vi "Launch Target Reply Time Test Actor.vi"   [LabVIEW 2023]
uses:
  Target Reply Time Test Actor/Target Reply Time Test Actor.lvclass
  Target Reply Time Test Actor/Target Reply Time Test Actor.lvclass/Target Reply Time Test Actor.ctl
  <vilib>/ni/Actors/Network Endpoint Actors/Protocols/Network Stream Strategy/Netowrk Stream Listener/Network Stream Listener.lvclass
  <vilib>/ActorFramework/Actor/Actor.lvclass
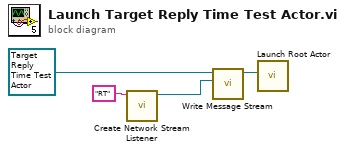
[diagram p0: block diagram]
diagram:
  n1 = call <vilib>:"Create Network Stream Listener.vi"("Name"="RT" ("Remote Name")) -> ("Network Stream Listener"=w3:refnum<class "Network Stream Listener.lvclass">)  [unwired: 10 in]
  n2 = call "Write Message Stream.vi"("Message Stream.lvclass"=w3, "Target Reply Time Test Actor in"=refnum<class "Target Reply Time Test Actor.lvclass"> refnum ("Target Reply Time Test Actor.lvlib:Target Reply Time Test Actor.lvclass")) -> ("Target Reply Time Test Actor out"=w4:refnum<class "Target Reply Time Test Actor.lvclass">)  [unwired: 9 in]
  n3 = call <vilib>:"Launch Root Actor.vi"("Actor"=w4) -> ()  [unwired: 9 in, 2 out]
